vi "User Console - Generate Transaction.vi"(8 "error in (no error)":errorcluster, 11 "Transactions":T2) -> (0 "error out":errorcluster, 2 "Transaction":T1)   [LabVIEW 2017]
uses:
  Controls/User Console - Transactions.ctl
  Controller/Controls/Controller Transaction.ctl
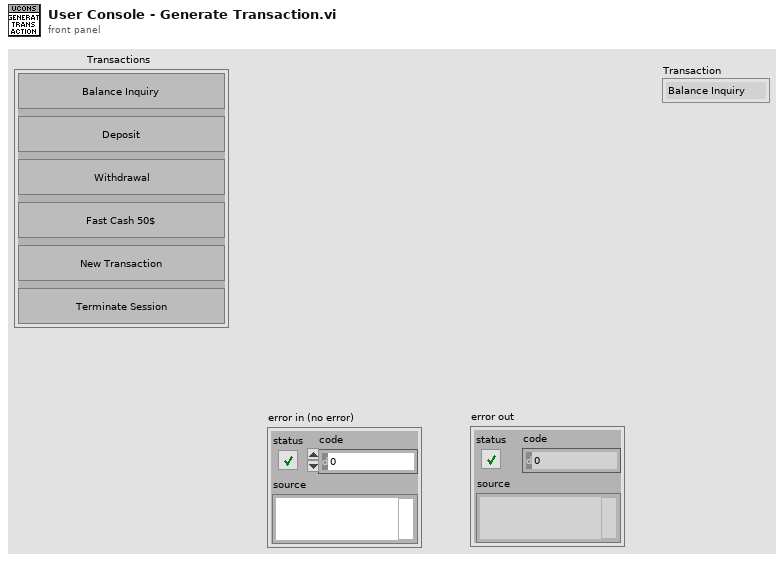
[diagram p1: front panel]
types:
  T1 = typedef "Controller Transaction.ctl" = enum16{"Balance Inquiry", "Deposit", "Withdrawal", "Fast Cash", "New Transaction", "Terminate Session"}
  T2 = typedef "User Console - Transactions.ctl" = cluster{"Balance Inquiry":bool, "Deposit":bool, "Withdrawal":bool, "Fast Cash":bool, "New Transaction":bool, "Terminate Session":bool}
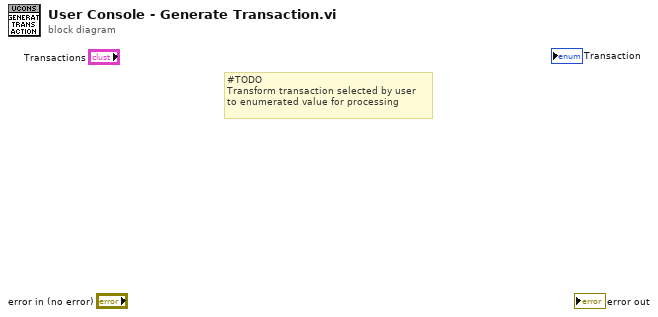
[diagram p0: block diagram]
diagram:
  # "#TODO\nTransform transaction selected by user\nto enumerated value for processing"
